vi "SENS_CORR_EXT_AUTO_PORT.vi"(0 "VISA IN":refnum<visa-resource-name>, 1 "Port":i32, 2 "ON/OFF":bool, 5 "error in":errorcluster, 7 "Channel":i32) -> (14 "VISA Out":refnum<visa-resource-name>, 19 "error out":errorcluster)   [LabVIEW 2018, in "PNA-X.lvlib"]
doc: "SENSe<cnum>:CORRection:EXTension:AUTO:PORT<n> <bool> \n(Read-Write) Enables and disables automatic port extensions on the specified port. \nParameters \n<cnum> Any existing channel number. If unspecified, value is set to 1 \n<n> PNA Port number to enable or disable for automatic port extensions. \n<bool> ON (or 1) - Enable \nOFF (or 0) - Disable \nExamples SENS:CORR:EXT:AUTO:PORT2 0 \nsense2:correction:extension:auto:port4 on \nQuery Syntax SENSe<cnum>:CORRection:EXTension:AUTO:PORT<n>? \nReturn Type Boolean \nDefault All ports ON (enabled)"
uses:
  PNA-X.lvlib
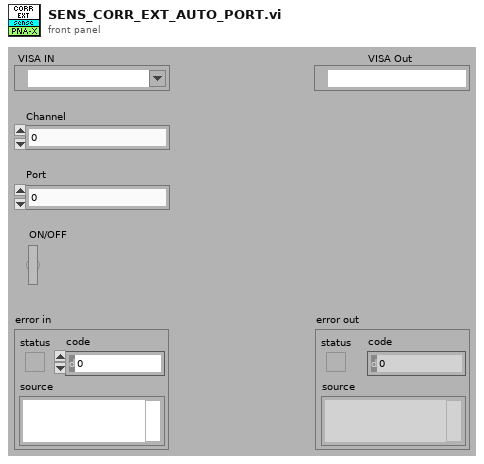
[diagram p1: front panel]
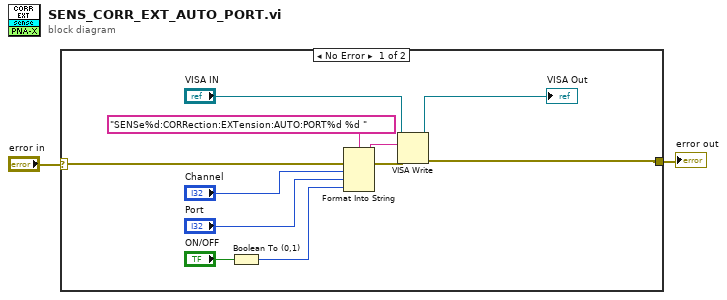
[diagram p0: block diagram]
diagram:
  n1 = case shown="No Error" "error in" {
    selector: "error in" -> [w13 w14]
    tunnel: [w8 w14] -> w1
    frame No Error {
      n2 = Boolean To (0,1)(Boolean="ON/OFF") -> (0, 1=w3:i16)
      n3 = Format Into String(format string="SENSe%d:CORRection:EXTension:AUTO:PORT%d %d " ("Cmdline"), error in=w13, "Channel", "Port", w3) -> (resulting string=w11:string, error out=w12:errorcluster)  [unwired: 1 in]
      n4 = VISA Write(VISA resource name="VISA IN", write buffer=w11, error in (no error)=w12) -> (VISA resource name out=→"VISA Out":refnum<visa-resource-name>, error out=w8:errorcluster)  [unwired: 1 out]
    }
    frame Error {
    }
  }
  "error out" <- w1
